vi "Init.MATLAB.vi"() -> (0 "reference":refnum<k24>)   [LabVIEW 2014]
uses:
  D:/Desktop/app/LabVIEW/MLApp.dll
  MLApp.dll
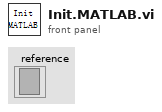
[diagram p1: front panel]
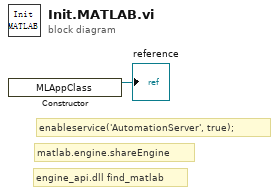
[diagram p0: block diagram]
diagram:
  # "engine_api.dll find_matlab"
  # "matlab.engine.shareEngine"
  # "enableservice('AutomationServer', true);"
  n1 = constructor class="MLAppClass"() -> (reference out=→"reference":refnum<k24>)  [unwired: 3 in, 2 out]
